vi "流程写入.vi"(11 "添加的路径":path) -> ()   [LabVIEW 2016, in "斯坦道氨氮.lvlib"]
uses:
  <vilib>/Utility/miscctls.llb/LVPointTypeDef.ctl
panel:
  in  "选项卡控件":enum32{"测试流程", "简易流程"}(tab)
  in  "量程下拉列表":enum16{"低量程", "高量程"}(ring)
  in  "水样测量":bool=TRUE
  in  "零点核查":bool
  in  "跨度核查":bool
  in  "标样核查":bool
  in  "加标回收":bool
  in  "简易流程":u16(ring) items=["注射泵复位"=0, "试剂填充"=1, "纯水填充"=2, "水样填充"=3, "标样核查标液填充(TN/TP)"=5, "零点核查标液填充"=6, "跨度核查标液填充"=7, "试剂管路清洗"=8, "总磷比色皿清洗"=9, "消解池清洗"=11, "注射器清洗"=12, "总磷LED灯值测试（纯水）"=13, "总磷LED灯值测试（水样）"=14, "高温高压阀测试"=18, "消解加热测试"=19, "总磷恒温测试"=20, "注射器恒温测试"=21, "管路排空"=24, "标样核查标液填充(TNTP)"=4, "总磷快捷显色测试（TNTP）"=22, "总磷快捷显色测试（TP）"=23]
  in  "关闭":bool
  out "字符串":string
  in  "写入":bool
  in  "参数下拉列表":u16(ring) items=["总磷"=1]
  # "请选择要写入的流程"
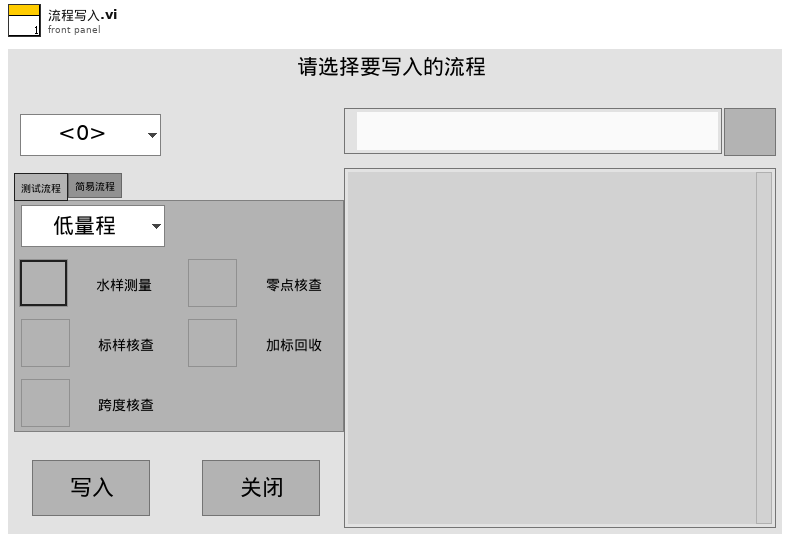
[diagram p1: front panel]
types:
  T1 = typedef "LVPointTypeDef.ctl" = cluster{"Horizontal":i16, "Vertical":i16}
  T2 = typedef "LVStringsAndValuesArrayTypeDef_U16.ctl" = cluster{"String":string, "Value":u16}[]
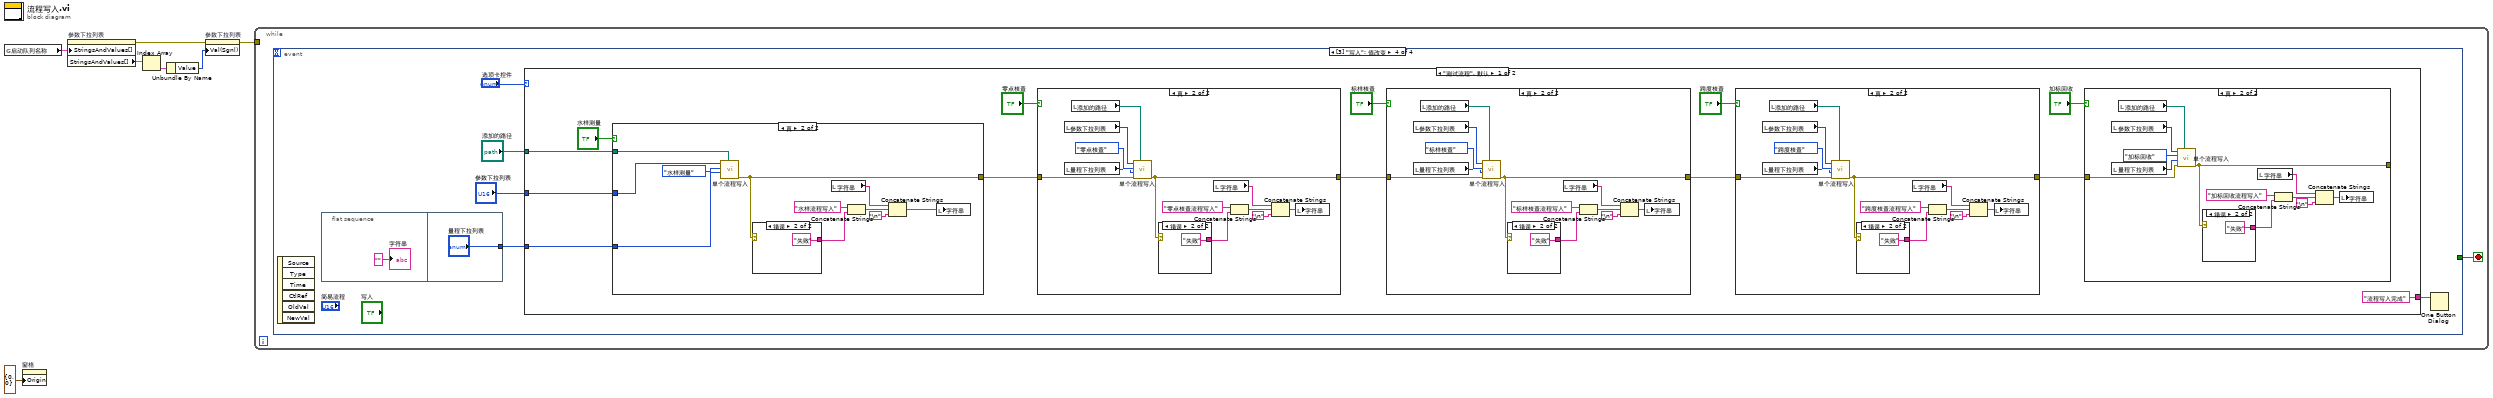
[diagram p0: block diagram]
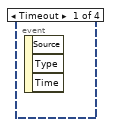
[diagram p2: hidden frame]
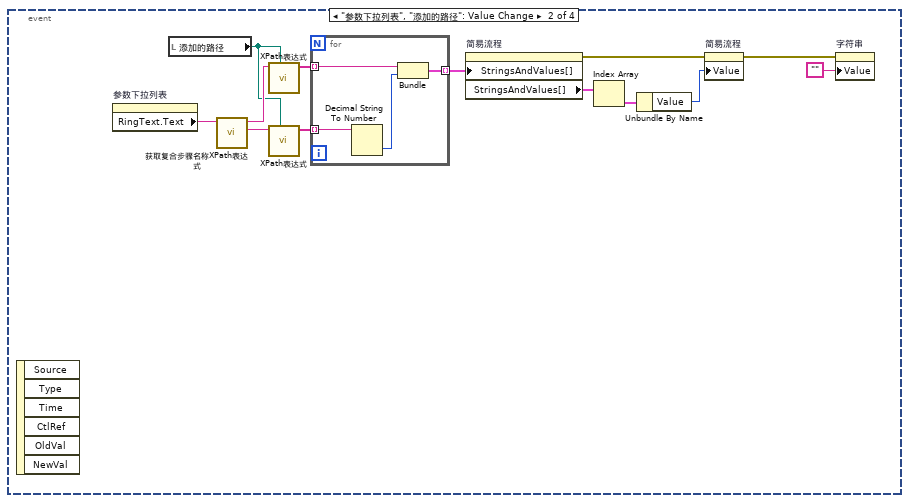
[diagram p3: hidden frame]
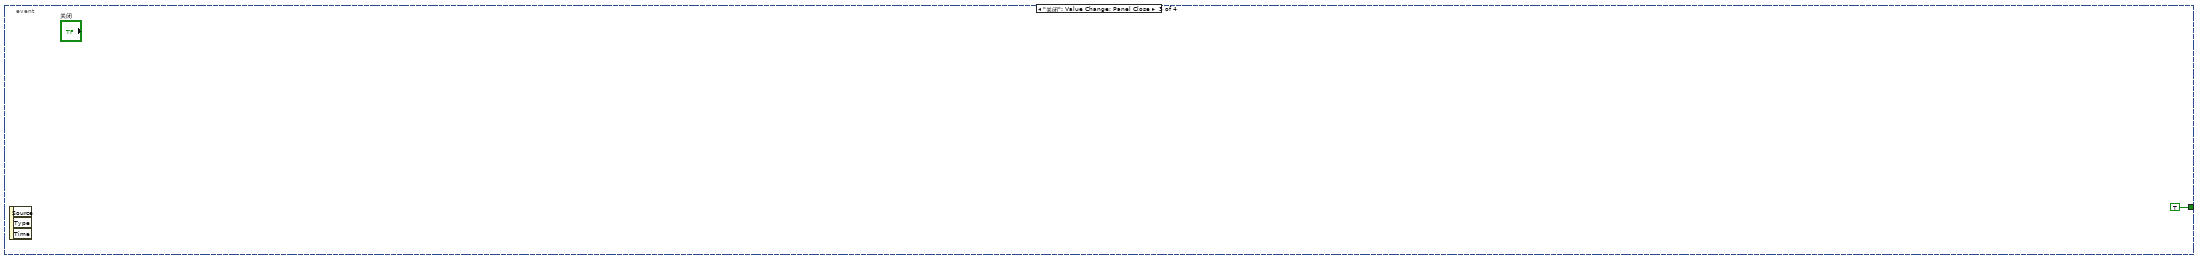
[diagram p4: hidden frame]
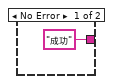
[diagram p6: hidden frame]
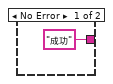
[diagram p8: hidden frame]
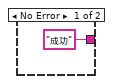
[diagram p10: hidden frame]
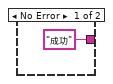
[diagram p12: hidden frame]
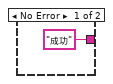
[diagram p14: hidden frame]
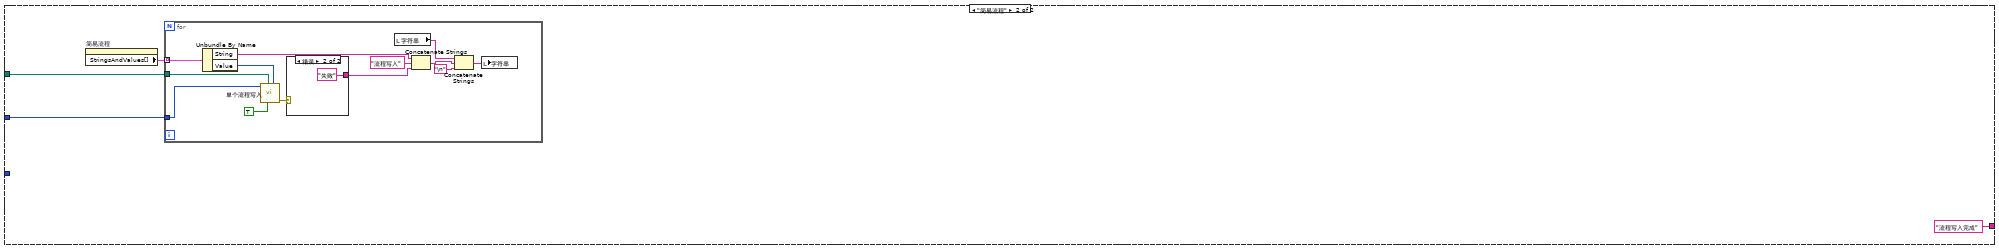
[diagram p15: hidden frame]
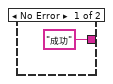
[diagram p16: hidden frame]
diagram:
  n1 = global read "总磷总氮断电保存全局变量.vi" "启动队列名称"() -> (w6:cluster{"String":string, "Value":u16}[])
  n2 = property on="窗格" class="Pane"("Origin"=T1 {"Horizontal"=0, "Vertical"=0} ("原点")) -> ()  [unwired: 2 in, 2 out]
  n3 = property on="参数下拉列表" class="Ring (严格)"("StringsAndValues[]"=w6) -> (error out=w5:errorcluster, "StringsAndValues[]"=w4:T2)  [unwired: 2 in, 1 out]
  n4 = Index Array(array=w4) -> (element=w3:cluster{"String":string, "Value":u16})  [unwired: 1 in]
  n5 = Unbundle By Name(w3) -> ("Value"=w2:u16)
  n6 = property on="参数下拉列表" class="Ring (严格)"(error in=w5, "Val(Sgnl)"=w2) -> (error out=w1:errorcluster)  [unwired: 1 in, 1 out]
  n7 = while {
    tunnel: w1 -> [_]
    stop <- w8 stop-if-true
    n8 = event shown="[3] \"写入\": 值改变" {
      selector: _ -> [_ _ _ _]
      dyn-events: _ -> [_ _ _ _]
      timeout: _ -> [_ _ _ _]
      tunnel: [_ _ TRUE _] -> w8
      event Timeout {
        n9 = event-data() -> ()  [unwired: 1 in, 3 out]
      }
      event "参数下拉列表", "添加的路径": Value Change {
        n10 = event-data() -> ()  [unwired: 1 in, 6 out]
        n11 = property on="参数下拉列表" class="Ring (严格)"() -> ("RingText.Text"=w20:string)  [unwired: 2 in, 2 out]
        n12 = local read "添加的路径"() -> (w19:path)
        n13 = call "获取复合步骤名称XPath表达式.vi"("查询参数"=w20) -> ("FlowId"=w18:string, "name"=w21:string)  [unwired: 9 in]
        n14 = call "XPath表达式.vi"("添加的路径"=w19, "XPath expression"=w21) -> ("数组"=w17:string[])  [unwired: 9 in]
        n15 = call "XPath表达式.vi"("添加的路径"=w19, "XPath expression"=w18) -> ("数组"=w16:string[])  [unwired: 9 in]
        n16 = for {
          tunnel: w17 -> [w25] mode=indexing
          tunnel: w16 -> [w24] mode=indexing
          tunnel: [w22] -> w15 mode=indexing
          n17 = Decimal String To Number(string=w24) -> (number=w23:i32)  [unwired: 2 in, 1 out]
          n18 = Bundle("node text"=w25, w23) -> (w22:cluster{"node text":string, i32})  [unwired: 1 in]
        }
        n19 = property on="简易流程" class="Ring (严格)"("StringsAndValues[]"=w15) -> (error out=w14:errorcluster, "StringsAndValues[]"=w13:T2)  [unwired: 2 in, 1 out]
        n20 = Index Array(array=w13) -> (element=w12:cluster{"String":string, "Value":u16})  [unwired: 1 in]
        n21 = Unbundle By Name(w12) -> ("Value"=w11:u16)
        n22 = property on="简易流程" class="Ring (严格)"(error in=w14, "Value"=w11) -> (error out=w10:errorcluster)  [unwired: 1 in, 1 out]
        n23 = property on="字符串" class="Str"(error in=w10, "Value"="") -> ()  [unwired: 1 in, 2 out]
      }
      event "关闭": Value Change; Panel Close {
        n24 = event-data() -> ()  [unwired: 1 in, 3 out]
      }
      event "写入": Value Change {
        n25 = event-data() -> ()  [unwired: 1 in, 6 out]
        n26 = flat-sequence {
          tunnel: ["量程下拉列表"] -> w30
          frame #0 {
            "字符串" <- ""
          }
          frame #1 {
          }
        }
        n27 = case shown="\"测试流程\", 默认" "选项卡控件" {
          tunnel: "参数下拉列表" -> [w44 w116]
          tunnel: w30 -> [w43 _]
          tunnel: "添加的路径" -> [w41 w117]
          tunnel: ["流程写入完成" ("消息") "流程写入完成" ("消息")] -> w27
          frame "测试流程", Default {
            n28 = case shown="真" "水样测量" {
              tunnel: w41 -> [_ w111]
              tunnel: w44 -> [_ w110]
              tunnel: w43 -> [_ w109]
              tunnel: [_ w107] -> w40
              frame False {
              }
              frame True {
                n29 = call "单个流程写入.vi"("添加的路径"=w111, "量程"=w109, "测量模式"=enum16{"水样测量", "零点核查", "跨度核查", "标样核查", "加标回收"}."水样测量", "测量参数"=w110) -> ("error out"=w107:errorcluster)  [unwired: 6 in, 1 out]
                n30 = case shown="错误" w107 {
                  tunnel: ["成功" "失败"] -> w104
                  frame No Error {
                  }
                  frame Error {
                  }
                }
                n31 = local read "字符串"() -> (w106:string)
                n32 = Concatenate Strings("水样流程写入", w104) -> (w103:string)
                n33 = Concatenate Strings(w106, w103, "\n") -> (w101:string)
                n34 = local write "字符串"(w101) -> ()
              }
            }
            n35 = case shown="真" "零点核查" {
              tunnel: [_ w97] -> w38
              tunnel: w40 -> [_ w87]
              frame False {
              }
              frame True {
                n36 = local read "参数下拉列表"() -> (w89:u16)
                n37 = local read "量程下拉列表"() -> (w88:enum16{"低量程", "高量程"})
                n38 = local read "添加的路径"() -> (w90:path)
                n39 = call "单个流程写入.vi"("添加的路径"=w90, "error in (no error)"=w87, "量程"=w88, "测量模式"=enum16{"水样测量", "零点核查", "跨度核查", "标样核查", "加标回收"}."零点核查", "测量参数"=w89) -> ("error out"=w97:errorcluster)  [unwired: 5 in, 1 out]
                n40 = case shown="错误" w97 {
                  tunnel: ["成功" "失败"] -> w94
                  frame No Error {
                  }
                  frame Error {
                  }
                }
                n41 = local read "字符串"() -> (w96:string)
                n42 = Concatenate Strings("零点核查流程写入", w94) -> (w93:string)
                n43 = Concatenate Strings(w96, w93, "\n") -> (w91:string)
                n44 = local write "字符串"(w91) -> ()
              }
            }
            n45 = case shown="真" "标样核查" {
              tunnel: [_ w83] -> w36
              tunnel: w38 -> [_ w73]
              frame False {
              }
              frame True {
                n46 = local read "参数下拉列表"() -> (w75:u16)
                n47 = local read "量程下拉列表"() -> (w74:enum16{"低量程", "高量程"})
                n48 = local read "添加的路径"() -> (w76:path)
                n49 = call "单个流程写入.vi"("添加的路径"=w76, "error in (no error)"=w73, "量程"=w74, "测量模式"=enum16{"水样测量", "零点核查", "跨度核查", "标样核查", "加标回收"}."标样核查", "测量参数"=w75) -> ("error out"=w83:errorcluster)  [unwired: 5 in, 1 out]
                n50 = case shown="错误" w83 {
                  tunnel: ["成功" "失败"] -> w80
                  frame No Error {
                  }
                  frame Error {
                  }
                }
                n51 = local read "字符串"() -> (w82:string)
                n52 = Concatenate Strings("标样核查流程写入", w80) -> (w79:string)
                n53 = Concatenate Strings(w82, w79, "\n") -> (w77:string)
                n54 = local write "字符串"(w77) -> ()
              }
            }
            n55 = case shown="真" "跨度核查" {
              tunnel: [_ w59] -> w33
              tunnel: w36 -> [_ w60]
              frame False {
              }
              frame True {
                n56 = local read "参数下拉列表"() -> (w62:u16)
                n57 = local read "量程下拉列表"() -> (w61:enum16{"低量程", "高量程"})
                n58 = local read "添加的路径"() -> (w63:path)
                n59 = call "单个流程写入.vi"("添加的路径"=w63, "error in (no error)"=w60, "量程"=w61, "测量模式"=enum16{"水样测量", "零点核查", "跨度核查", "标样核查", "加标回收"}."跨度核查", "测量参数"=w62) -> ("error out"=w59:errorcluster)  [unwired: 5 in, 1 out]
                n60 = case shown="错误" w59 {
                  tunnel: ["成功" "失败"] -> w67
                  frame No Error {
                  }
                  frame Error {
                  }
                }
                n61 = local read "字符串"() -> (w69:string)
                n62 = Concatenate Strings("跨度核查流程写入", w67) -> (w66:string)
                n63 = Concatenate Strings(w69, w66, "\n") -> (w64:string)
                n64 = local write "字符串"(w64) -> ()
              }
            }
            n65 = case shown="真" "加标回收" {
              tunnel: [_ w55] -> _
              tunnel: w33 -> [_ w45]
              frame False {
              }
              frame True {
                n66 = local read "参数下拉列表"() -> (w47:u16)
                n67 = local read "量程下拉列表"() -> (w46:enum16{"低量程", "高量程"})
                n68 = local read "添加的路径"() -> (w48:path)
                n69 = call "单个流程写入.vi"("添加的路径"=w48, "error in (no error)"=w45, "量程"=w46, "测量模式"=enum16{"水样测量", "零点核查", "跨度核查", "标样核查", "加标回收"}."加标回收", "测量参数"=w47) -> ("error out"=w55:errorcluster)  [unwired: 5 in, 1 out]
                n70 = case shown="错误" w55 {
                  tunnel: ["成功" "失败"] -> w52
                  frame No Error {
                  }
                  frame Error {
                  }
                }
                n71 = local read "字符串"() -> (w54:string)
                n72 = Concatenate Strings("加标回收流程写入", w52) -> (w51:string)
                n73 = Concatenate Strings(w54, w51, "\n") -> (w49:string)
                n74 = local write "字符串"(w49) -> ()
              }
            }
          }
          frame "简易流程" {
            n75 = property on="简易流程" class="Ring (严格)"() -> ("StringsAndValues[]"=w115:T2)  [unwired: 2 in, 2 out]
            n76 = for {
              tunnel: w115 -> [w120] mode=indexing
              tunnel: w117 -> [w123]
              tunnel: w116 -> [w122]
              n77 = Unbundle By Name(w120) -> ("String"=w119:string, "Value"=w118:u16)
              n78 = call "单个流程写入.vi"("简易流程Id"=w118, "是否是简易流程"=TRUE, "添加的路径"=w123, "测量参数"=w122) -> ("error out"=w130:errorcluster)  [unwired: 6 in, 1 out]
              n79 = case shown="错误" w130 {
                tunnel: ["成功" "失败"] -> w127
                frame No Error {
                }
                frame Error {
                }
              }
              n80 = local read "字符串"() -> (w129:string)
              n81 = Concatenate Strings(w119, "流程写入", w127) -> (w126:string)
              n82 = Concatenate Strings(w129, w126, "\n") -> (w124:string)
              n83 = local write "字符串"(w124) -> ()
            }
          }
        }
        n84 = One Button Dialog(message=w27) -> ()  [unwired: 1 in, 1 out]
      }
    }
  }
